vi "Siglent SDG X Series Standard Waveform.vi"() -> ()   [LabVIEW 2022 SP3]
doc: "This example shows how to generate a standard waveform."
uses:
  Siglent SDG X Series.lvlib
panel:
  in  "Amplitude (1.0 Vpp)":dbl=1.0 format="%#.3f"
  in  "VISA resource name":refnum<visa-resource-name>
  in  "DC Offset (0.00 V)":dbl
  in  "Frequency (1000 Hz)":dbl=1000.0 format="%#.6g"
  in  "Channel (1:Channel 1)":i32(ring)=1 items=["Channel 1"=1, "Channel 2"=2]
  in  "Waveform Function (0: Sine)":u16(ring) items=["Sine", "Square", "Triangle", "DC", "Pulse", "Arb"]
  # "(c) 2017 SIGLENT TECHNOLOGIES CO.,LTD. ALL RIGHTS RESERVED."
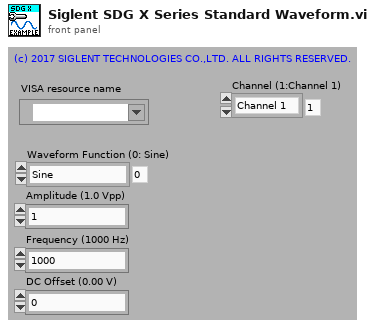
[diagram p1: front panel]
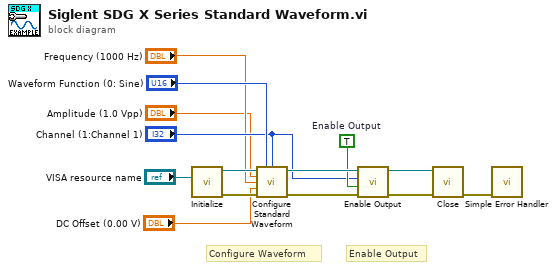
[diagram p0: block diagram]
diagram:
  w7 = TRUE  # Enable Output
  # "Enable Output"
  # "Configure Waveform"
  n1 = call "Initialize.vi"("VISA resource name"="VISA resource name") -> ("error out"=w13:errorcluster, "VISA resource name out"=w14:refnum<visa-resource-name>)  [unwired: 9 in]
  n2 = call "Configure Standard Waveform.vi"("VISA resource name"=w14, "Waveform Function (0: Sine)"="Waveform Function (0: Sine)", "Channel (1:Channel 1)"="Channel (1:Channel 1)", "Amplitude (1.0 Vpp)"="Amplitude (1.0 Vpp)", "Frequency (1000 Hz)"="Frequency (1000 Hz)", "DC Offset (0.00 V)"="DC Offset (0.00 V)", "error in (no error)"=w13) -> ("VISA resource name out"=w11:refnum<visa-resource-name>, "error out"=w10:errorcluster)  [unwired: 7 in]
  n3 = call "Enable Output.vi"("error in (no error)"=w10, "Enable Output (T: Enable)"=w7, "Channel (1:Channel 1)"="Channel (1:Channel 1)", "VISA resource name"=w11) -> ("error out"=w8:errorcluster, "VISA resource name out"=w9:refnum<visa-resource-name>)  [unwired: 6 in]
  n4 = call "Close.vi"("error in (no error)"=w8, "VISA resource name"=w9) -> ("error out"=w12:errorcluster)  [unwired: 9 in]
  n5 = call <vilib>:"Simple Error Handler.vi"("error in (no error)"=w12) -> ()  [unwired: 4 in, 5 out]
